vi "Insert Named Instr.vi"(0 "new instrument":T1, 1 "Setup":T2[](array[typedef]) {"Private"."Offset" format="%^_3e"; "Private"."Scale Factors" format="%^_3e"}, 2 "Configured Names":string[](array[string]), 3 "Instrument List":i32) -> (5 "dup Setup":T2[](array[typedef]) {"Private"."Offset" format="%^_3e"; "Private"."Scale Factors" format="%^_3e"}, 7 "Item Names":string[](array[string]), 8 "Instrument List Out":i32)   [LabVIEW 2019]
uses:
  Sub Controls/Instrument Properties.ctl
  Sub Controls/Public.ctl
  Sub Controls/Private.ctl
  Sub Controls/Instrument Ref.ctl
  Sub Controls/SystemCheckBox-resize.ctl
  Sub Controls/Instrument Info.ctl
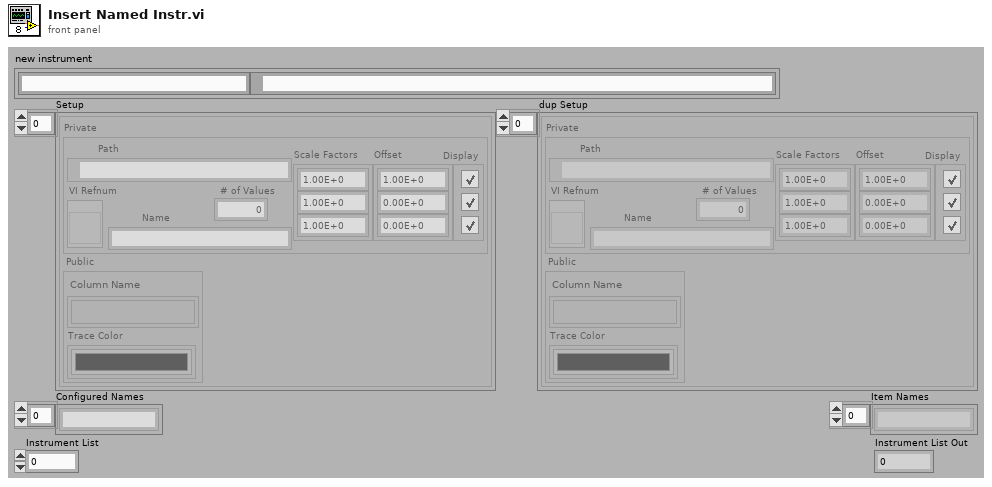
[diagram p1: front panel]
types:
  T1 = typedef "Instrument Info.ctl" = cluster{"Name":string, "path":path}
  T2 = typedef "Instrument Properties.ctl" = cluster{"Public":T3, "Private":T4}
  T3 = typedef "Public.ctl" = cluster{"Column Name":string[], "Trace Color":u32[]}
  T4 = typedef "Private.ctl" = cluster{"Path":path, "VI Refnum":T5, "Name":string, "# of Values":i32, "Scale Factors":dbl[], "Display":T6[], "Offset":dbl[]}
  T5 = typedef "Instrument Ref.ctl" = refnum<vi>
  T6 = typedef "SystemCheckBox-resize.ctl" = bool
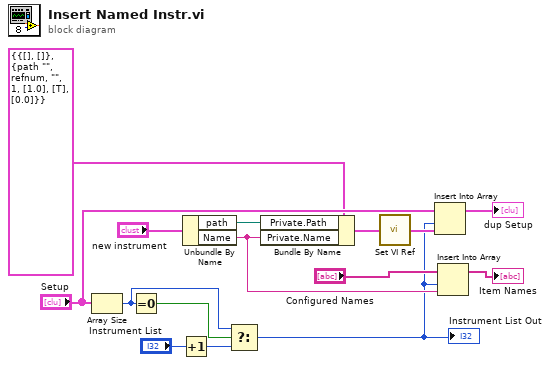
[diagram p0: block diagram]
diagram:
  n1 = Array Size(array="Setup") -> (size(s)=w2:i32)
  n2 = Equal To 0?(x=w2) -> (x = 0?=w3:bool)
  n3 = Increment(x="Instrument List") -> (x+1=w12:i32)
  n4 = Unbundle By Name("new instrument") -> ("path"=w7:path, "Name"=w6:string)
  n5 = Select(t=w2, s=w3, f=w12) -> (s? t:f=w5:i32)
  "Instrument List Out" <- w5
  n6 = Bundle By Name(cluster=T2 {"Public"={"Column Name"=[], "Trace Color"=[]}, "Private"={"Path"=path "", "VI Refnum"=refnum, "Name"="", "# of Values"=1, "Scale Factors"=[1.0], "Display"=[TRUE], "Offset"=[0.0]}} ("Instrument Prop"), "Private.Path"=w7, "Private.Name"=w6) -> (w11:T2)
  n7 = call "Set VI Ref.vi"("Instrument Prop In"=w11) -> ("Instrument Prop Out"=w10:T2)
  n8 = Insert Into Array(array="Setup", index=w5, new element=w10) -> (→"dup Setup":T2[])
  n9 = Insert Into Array(array="Configured Names", index=w5, new element=w6) -> (→"Item Names":string[])
